vi "getIP.vi"(8 "error in (no error)":errorcluster, 11 "ElectrometerController in":refnum<class "ElectrometerController.lvclass">) -> (0 "error out":errorcluster, 2 "name":string, 3 "ElectrometerController out":refnum<class "ElectrometerController.lvclass">)   [LabVIEW 2016, in "ElectrometerController.lvclass"]
uses:
  ElectrometerController.lvclass
panel:
  out "net address":u32
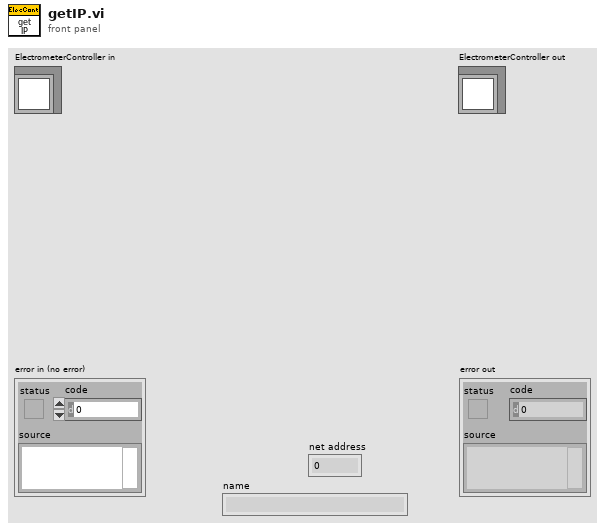
[diagram p1: front panel]
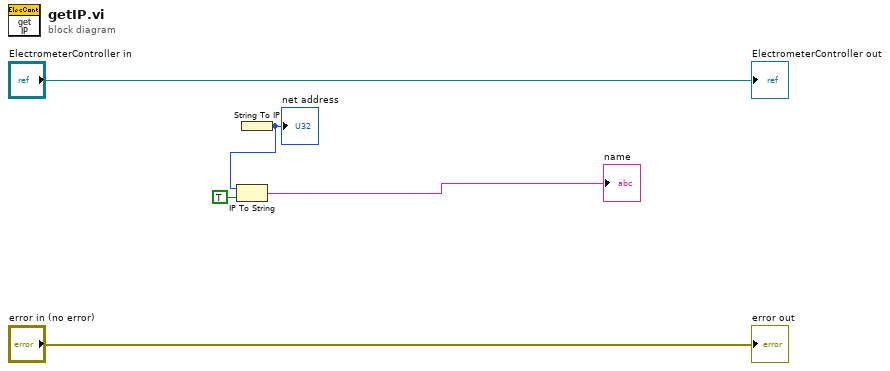
[diagram p0: block diagram]
diagram:
  n1 = String To IP() -> (0:w2:u32)  [unwired: 1 in]
  "net address" <- w2
  n2 = IP To String(1:TRUE ("dot notation? (F)"), 2:w2) -> (0:→"name":string)
  "error out" <- "error in (no error)"
  "ElectrometerController out" <- "ElectrometerController in"
